vi "Save Calibration File.vi"(8 "error in":errorcluster, 9 "Calibration Values":string, 10 "File Name":string, 11 "Cali File Path":path=path "C:/Users/scholp/Desktop/Calibration .txt files/Calibration Values.txt") -> (0 "error out":errorcluster)   [LabVIEW 2020, in "SubVIs.lvlib"]
uses:
  SubVIs.lvlib
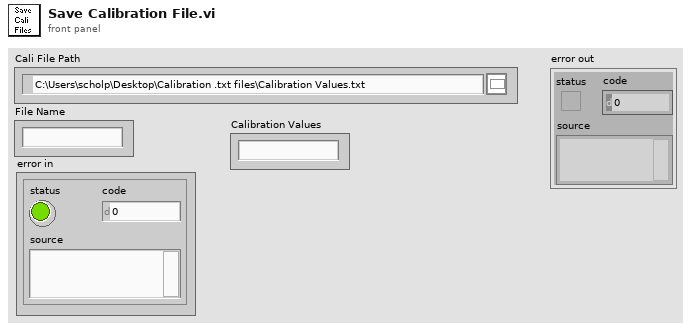
[diagram p1: front panel]
types:
  T1 = enum16{"open", "replace", "create", "open or create", "replace or create", "replace or create with confirmation"}
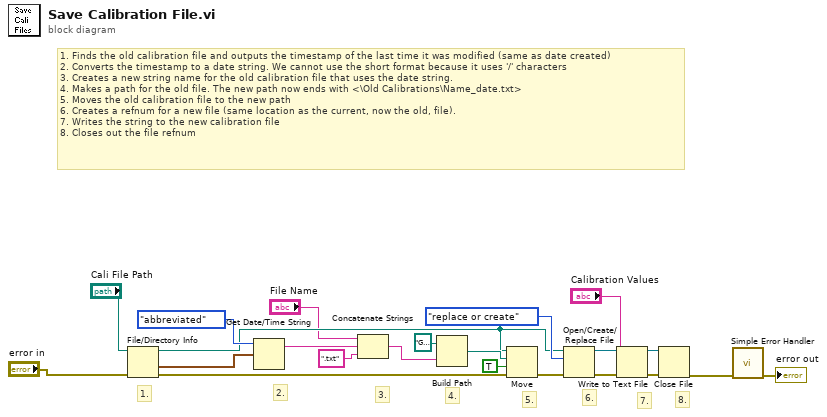
[diagram p0: block diagram]
diagram:
  # "1. Finds the old calibration file and outputs the timestamp of the last time it was modified (same as date created)\n2. Converts the timestamp to a date string. We cannot use the short format because it uses '/' characters\n3. Creates a new string name for the old calibration file that uses the date string.\n4. Makes a path for the old file. The new path now ends with <\\Old Calibrations\\Name_date.txt>\n5. Moves the old calibration file to the new path\n6. Creates a refnum for a new file (same location as the current, now the old, file).\n7. Writes the string to the new calibration file\n8. Closes out the file refnum"
  # "8."
  # "7."
  # "6."
  # "5."
  # "4."
  # "3."
  # "2."
  # "1."
  n1 = File/Directory Info(path="Cali File Path", error in="error in") -> (path out=w7:path, last mod=w10:timestamp, error out=w12:errorcluster)  [unwired: 4 out]
  n2 = Get Date/Time String(date format (0)=enum16{"short", "long", "abbreviated"}."abbreviated", seconds (now)=w10) -> (date string=w9:string)  [unwired: 1 in, 1 out]
  n3 = Concatenate Strings("File Name", w9, ".txt" ("string")) -> (w14:string)
  n4 = Build Path(base path=path "G:/1-Booth Program Updated - 2019/Calibration Files/Old Calibrations" ("target path (use dialog)"), name or relative path=w14) -> (appended path=w17:path)
  n5 = Move(source path=w7, error in=w12, 9:TRUE ("overwrite (F)"), 10:w17) -> (error out=w18:errorcluster)  [unwired: 1 in, 2 out]
  n6 = Open/Create/Replace File(file path (use dialog)=w7, error in=w18, operation (0:open)=T1."replace or create") -> (refnum out=w21:refnum<file>, error out=w13:errorcluster)  [unwired: 3 in, 1 out]
  n7 = Write to Text File(file (use dialog)=w21, text="Calibration Values", error in=w13) -> (refnum out=w20:refnum<file>, error out=w22:errorcluster)  [unwired: 1 in, 1 out]
  n8 = Close File(refnum=w20, error in=w22) -> (error out=w4:errorcluster)  [unwired: 1 out]
  n9 = call <vilib>:"Simple Error Handler.vi"("error in (no error)"=w4) -> ("error out"=→"error out":errorcluster)  [unwired: 4 in, 4 out]
